vi "Test1.vi"() -> ()   [LabVIEW 2016]
panel:
  out "call chain":string[](array[string])
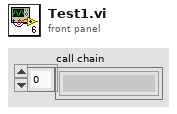
[diagram p1: front panel]
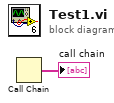
[diagram p0: block diagram]
diagram:
  n1 = Call Chain() -> (call chain=→"call chain":string[])
